vi "Add Available Measurement.vi"(8 "error in (no error)":errorcluster, 10 "Measurement.lvclass":refnum<class "Measurement.lvclass">, 11 "Controller in":refnum<class "Controller.lvclass">) -> (0 "error out":errorcluster, 3 "Controller out":refnum<class "Controller.lvclass">)   [LabVIEW 2026, in "Controller Actor.lvlib" / "Controller.lvclass"]
uses:
  Controller.lvclass
  C:/Program Files/National Instruments/LabVIEW 2026/vi.lib/ActorFramework/Actor/Actor.lvclass
  Measurement Actor/Measurement.lvclass
  Controller.lvclass/Controller.ctl
  Extensible-Config-Dialog/Configuration.lvclass/Configuration.ctl
  Measurement Actor/Measurement.lvclass/Measurement.ctl
  <vilib>/ActorFramework/Actor/Actor.lvclass/Actor.ctl
  <vilib>/ActorFramework/Message Enqueuer/Message Enqueuer.lvclass/Message Enqueuer.ctl
  <vilib>/ActorFramework/Message Enqueuer/Init from Existing Queue.vi
  Measurement Actor/Configuration/Step Configuration.lvclass
  C:/Users/E2013170/Documents/GitHub/Measurement-Utility-Reference/components/Extensible-Config-Dialog/Configuration.lvclass
  Extensible-Config-Dialog/Configuration.lvclass
  <vilib>/ActorFramework/Message Enqueuer/Message Enqueuer.lvclass
  Messages/Log Status/Log Status.lvclass
  <vilib>/ActorFramework/Actor/Actor.lvclass
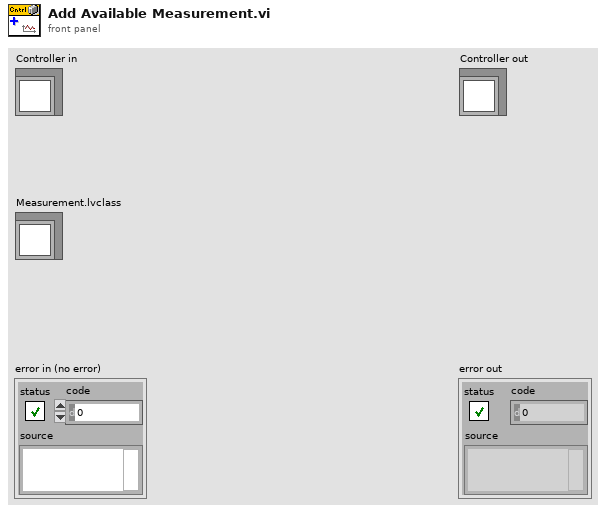
[diagram p1: front panel]
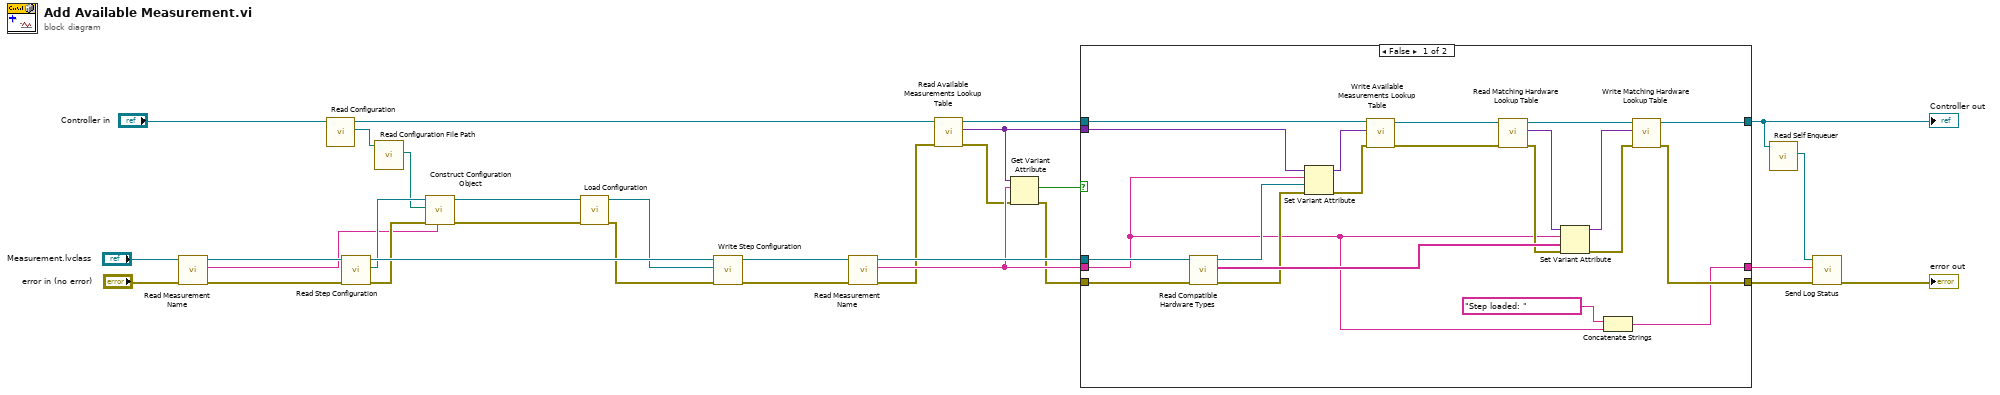
[diagram p0: block diagram]
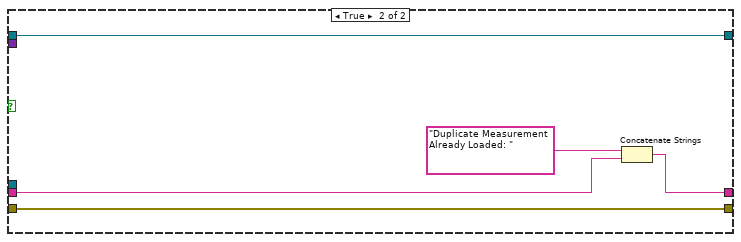
[diagram p2: hidden frame]
diagram:
  n1 = call "Read Measurement Name.vi"("error in (no error)"="error in (no error)", "Measurement in"="Measurement.lvclass") -> ("error out"=w2:errorcluster, "Measurement Name"=w1:string, "Measurement out"=w3:refnum<class "Measurement.lvclass">)  [unwired: 7 in]
  n2 = call "Read Configuration.vi"("Controller in"="Controller in") -> ("Configuration.lvlib:Configuration.lvclass"=w7:refnum<class "Configuration.lvclass">, "Controller out"=w17:refnum<class "Controller.lvclass">)  [unwired: 8 in, 1 out]
  n3 = call "Read Step Configuration.vi"("error in (no error)"=w2, "Measurement in"=w3) -> ("error out"=w9:errorcluster, "Measurement Actor.lvlib:Step Configuration.lvclass"=w13:refnum<class "Step Configuration.lvclass">, "Measurement out"=w14:refnum<class "Measurement.lvclass">)  [unwired: 7 in]
  n4 = call "Read Configuration File Path.vi"("Configuration in"=w7) -> ("Configuration File Path"=w6:path)  [unwired: 8 in, 2 out]
  n5 = call "Construct Configuration Object.vi"("Group Name"=w1, "error in (no error)"=w9, "Configuration File Path"=w6, "Configuration in"=w13) -> ("error out"=w10:errorcluster, "Configuration out"=w11:refnum<class "Step Configuration.lvclass">)  [unwired: 4 in, 2 out]
  n6 = call "Load Configuration.vi"("error in (no error)"=w10, "Configuration in"=w11) -> ("error out"=w8:errorcluster, "Configuration out"=w12:refnum<class "Step Configuration.lvclass">)  [unwired: 7 in, 1 out]
  n7 = call "Write Step Configuration.vi"("error in (no error)"=w8, "Measurement Actor.lvlib:Step Configuration.lvclass"=w12, "Measurement in"=w14) -> ("error out"=w15:errorcluster, "Measurement out"=w16:refnum<class "Measurement.lvclass">)  [unwired: 7 in]
  n8 = call "Read Measurement Name.vi"("error in (no error)"=w15, "Measurement in"=w16) -> ("error out"=w25:errorcluster, "Measurement Name"=w26:string, "Measurement out"=w29:refnum<class "Measurement.lvclass">)  [unwired: 7 in]
  n9 = call "Read Available Measurements Lookup Table.vi"("error in (no error)"=w25, "Controller in"=w17) -> ("error out"=w24:errorcluster, "Available Measurements Lookup Table"=w22:variant, "Controller out"=w28:refnum<class "Controller.lvclass">)  [unwired: 7 in]
  n10 = Get Variant Attribute(Variant=w22, name=w26, error in=w24) -> (found=w27:bool, error out=w23:errorcluster)  [unwired: 1 in, 2 out]
  n11 = case shown="False" w27 {
    tunnel: [w32 w54] -> w30
    tunnel: [w37 w56] -> w20
    tunnel: w28 -> [w51 w56]
    tunnel: w29 -> [w50 _]
    tunnel: w23 -> [w35 w54]
    tunnel: w26 -> [w34 w53]
    tunnel: w22 -> [w33 _]
    tunnel: [w31 w52] -> w19
    frame False {
      n12 = call-dynamic "Read Compatible Hardware Types.vi"("error in (no error)"=w35, "Measurement in"=w50) -> ("error out"=w42:errorcluster, "Compatible Hardware Types"=w48:string[], "Measurement out"=w43:refnum<class "Measurement.lvclass">)  [unwired: 7 in]
      n13 = Set Variant Attribute(Variant=w33, name=w34, value=w43, error in=w42) -> (Variant out=w49:variant, error out=w41:errorcluster)  [unwired: 1 out]
      n14 = call "Write Available Measurements Lookup Table.vi"("error in (no error)"=w41, "Available Measurements Lookup Table"=w49, "Controller in"=w51) -> ("error out"=w40:errorcluster, "Controller out"=w45:refnum<class "Controller.lvclass">)  [unwired: 7 in]
      n15 = call "Read Matching Hardware Lookup Table.vi"("error in (no error)"=w40, "Controller in"=w45) -> ("error out"=w39:errorcluster, "Matching Hardware Lookup Table"=w47:variant, "Controller out"=w46:refnum<class "Controller.lvclass">)  [unwired: 7 in]
      n16 = Set Variant Attribute(Variant=w47, name=w34, value=w48, error in=w39) -> (Variant out=w44:variant, error out=w38:errorcluster)  [unwired: 1 out]
      n17 = Concatenate Strings("Step loaded: " ("string"), w34) -> (w31:string)
      n18 = call "Write Matching Hardware Lookup Table.vi"("error in (no error)"=w38, "Matching Hardware Lookup Table"=w44, "Controller in"=w46) -> ("error out"=w32:errorcluster, "Controller out"=w37:refnum<class "Controller.lvclass">)  [unwired: 7 in]
    }
    frame True {
      n19 = Concatenate Strings("Duplicate Measurement Already Loaded: " ("string"), w53) -> (w52:string)
    }
  }
  "error out" <- w30
  "Controller out" <- w20
  n20 = call <vilib>:"Read Self Enqueuer.vi"("Actor"=w20) -> ("Self Enqueuer"=w21:refnum<class "Message Enqueuer.lvclass">)  [unwired: 10 in]
  n21 = call "Send Log Status.vi"("String"=w19, "Message Enqueuer in"=w21) -> ()  [unwired: 8 in, 2 out]
